vi "Disconnect.vi"(8 "error in (no error)":errorcluster, 11 "Videoscan in":refnum<class "Videoscan.lvclass">) -> (0 "error out":errorcluster, 3 "Videoscan out":refnum<class "Videoscan.lvclass">)   [LabVIEW 2014, in "Videoscan.lvclass"]
uses:
  Videoscan.lvclass
  Videoscan.lvclass/Videoscan.ctl
  VideoScanLibrary/VideoScanDeviceLibrary.lvclass
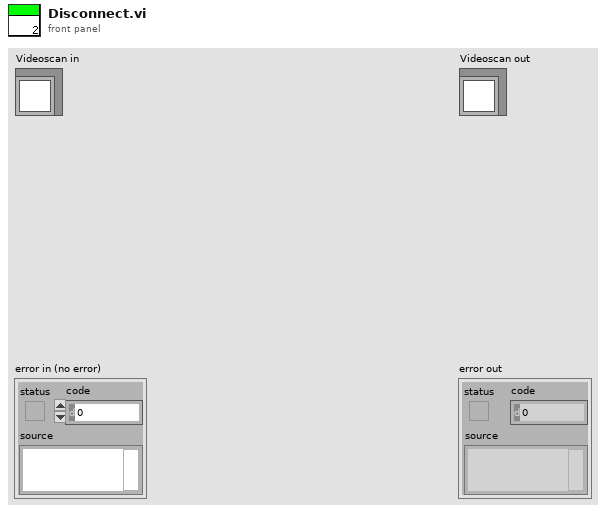
[diagram p1: front panel]
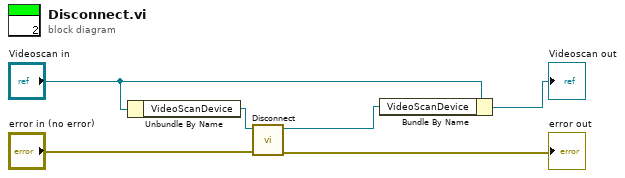
[diagram p0: block diagram]
diagram:
  n1 = Unbundle By Name("Videoscan in") -> ("VideoScanDevice"=w3:refnum<class "VideoScanDeviceLibrary.lvclass">)
  n2 = call "Disconnect.vi"("error in (no error)"="error in (no error)", "VideoScanCamera in"=w3) -> ("error out"=→"error out":errorcluster, "VideoScanCamera out"=w4:refnum<class "VideoScanDeviceLibrary.lvclass">)  [unwired: 8 in]
  n3 = Bundle By Name(cluster="Videoscan in", "VideoScanDevice"=w4) -> (→"Videoscan out":refnum<class "Videoscan.lvclass">)
